vi "Untitled 4.vi"() -> ()   [LabVIEW 2016]
uses:
  <vilib>/addons/database/NI_Database_API.lvlib
  <vilib>/addons/database/Connection.llb/Conn Execute.vi
  <vilib>/addons/database/Recordset.llb/Rec Destroy - Connection.vi
panel:
  in  "POMPA":T1 {"DIAM mand [mm]" items=["--", "15", "20", "25", "27", "32", "40", "50", "65", "80", "100", "125", "150"]; "DIAM asp [mm]" items=["--", "15", "20", "25", "27", "32", "40", "50", "65", "80", "100", "125", "150"]; "MODELLO" items=["TECH 2", "TECH 3", "1", "2", "3", "4", "5", "1- FLOOR", "2- FLOOR", "2- VORTEX", "3- VORTEX", "2/20", "3/20", "4/40", "5/40", "TR 075", "30/50", "3SR2-15", "3SR2-22", "3SR2-30", "3SR2-43", "44/8", "4/9", "4/7", "4/14", "4/6 - 60Hz", "------", "12/6", "40/35", "55/35", "75/35", "40/65", "55/65", "75/65", "40/100", "50/100", "55/100", "15-50_st", "10-45", "15/50", "20/50", "30/50", "40/50", "50/50", "55/50", "TRm 1.1", "TRm 2.2", "18/18"]; "FAMIGLIA" items=["--", "TOP", "RX", "VX-71", "BC-71", "D", "VXC-71", "MC-71", "DC", "TRITUS", "VXC-80", "MC-80", "NK", "UP", "DAVIS", "4BLOCK", "4SR", "6SR", "TOP MULTI", "VXC4", "BC-100", "VX-100", "3SR", "4BLOCK", "MC4"]}
  in  "DATI GENERALI":T2 {"SCOPO" items=["--", "Audit", "Prototipo", "Campionatura", "Preserie", "Qualità", "Rientri", "Concorrenza"]; "NORMA DI RIFERIMENTO" items=["--", "0", "1", "2"]}
  in  "MOTORE":T3 {"GRADO IP" items=["--", "23", "44", "55", "68", "X4", "X5", "X8"]; "CLASSE ISOLAMENTO" items=["--", "B", "F", "H"]; "CONDENSATORE [uF,V]" items=["1", "2", "6.3", "8", "10", "12.5", "14", "16", "20", "25", "31.5", "35", "45", "------", "50"]; "Frequenza" items=["--", "50", "60", "Variabile"]; "FASI" items=["--", "Trifase", "Monofase"]; "MEC" items=["--", "56", "63", "71", "80", "90", "100", "112", "132", "160", "200", "250"]; "STATO" items=["--", "STD", "Prototipo", "Concorrenza"]}
  in  "CONDIZIONI DI PROVA":T4 {"COLLAUDATORE" items=["--", "CREMONESE G.PIETRO"]; "Fluido" items=["--", "Acqua"]}
  out "BOLLETTINO CARICATO":T5
  out "reversed":string
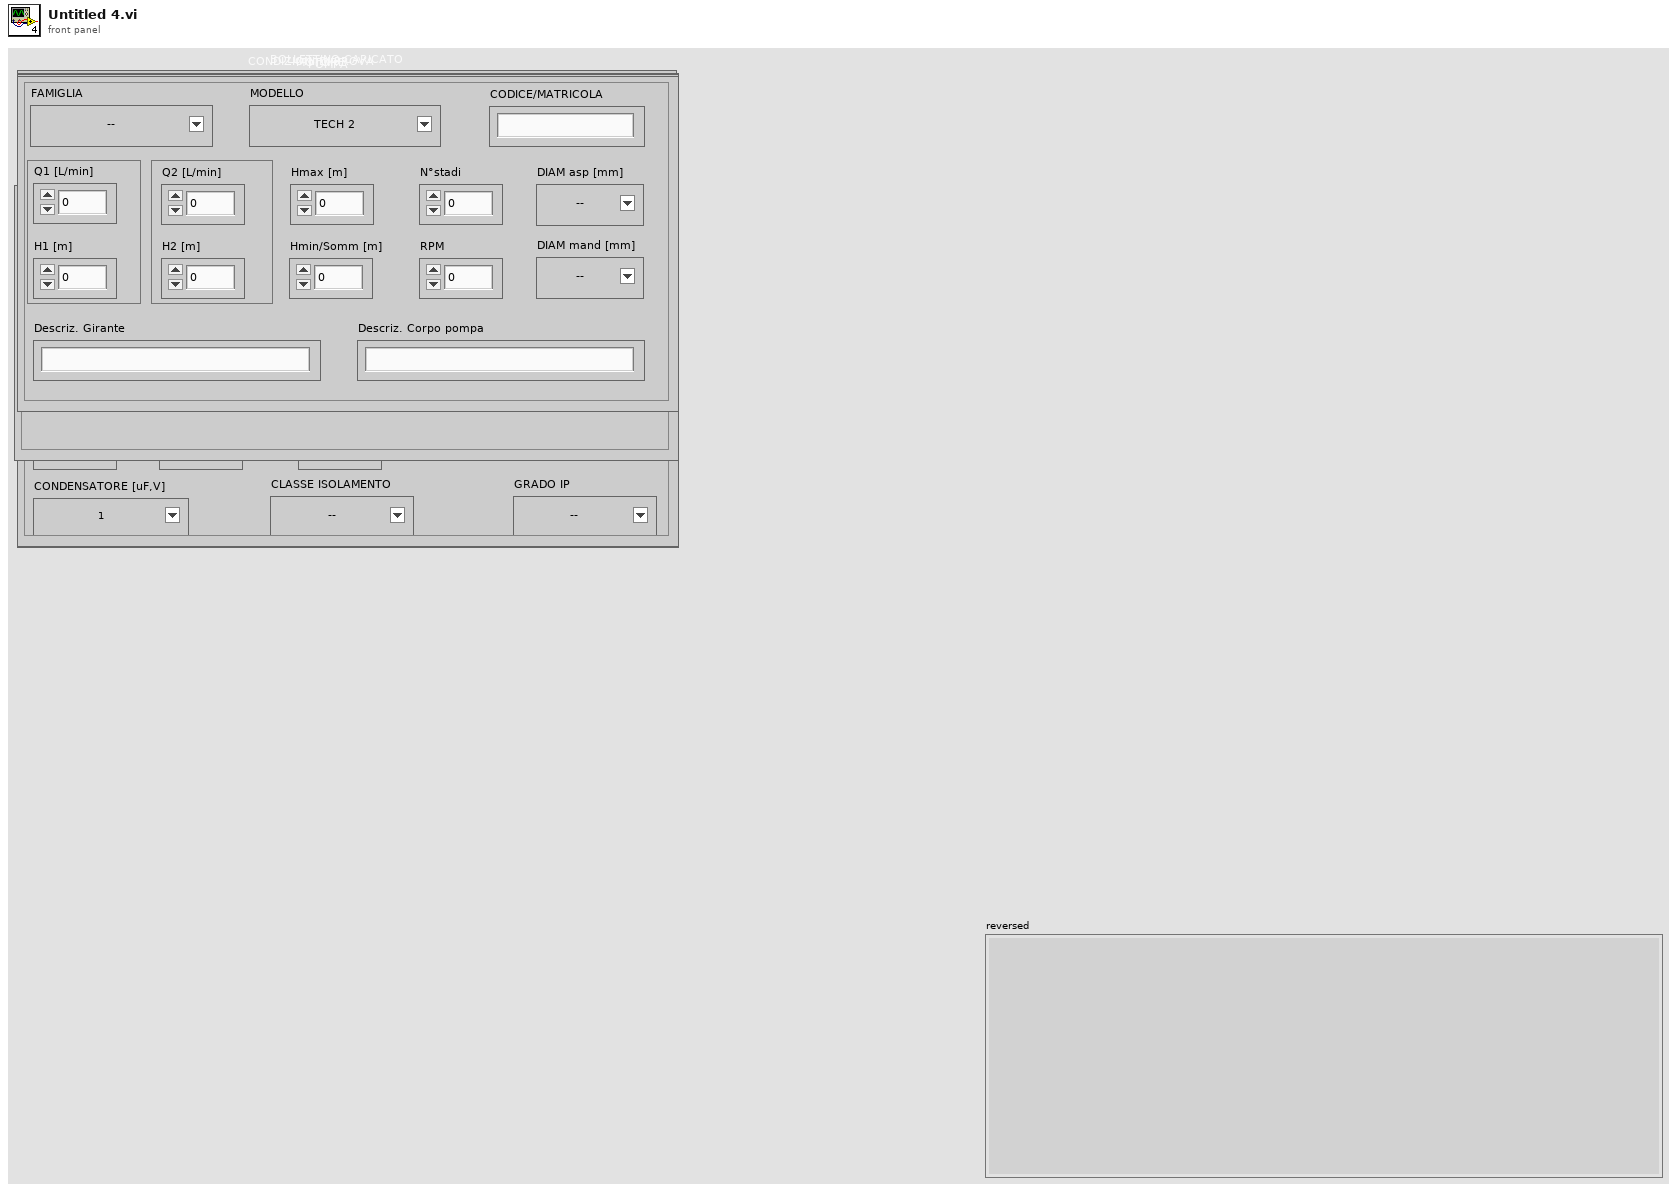
[diagram p1: front panel]
types:
  T1 = cluster{"FAMIGLIA":u16, "MODELLO":u16, "CODICE/MATRICOLA":string, "Q1 [L/min]":dbl, "Q2 [L/min] ":dbl, "H1 [m]":dbl, "H2 [m]":dbl, "Hmax [m]":dbl, "Hmin/Somm [m]":dbl, "RPM":dbl, "N°stadi":dbl, "DIAM asp [mm]":u16, "DIAM mand [mm]":u16, "Descriz. Girante":string, "Descriz. Corpo pompa":string}
  T2 = cluster{"NORMA DI RIFERIMENTO":u16, "SCOPO":u16, "ID PROGETTO":string, "N°ORDINE/PLP":string, "RIF/CLIENTE":string}
  T3 = cluster{"MODELLO E TIPO":string, "STATO":u16, "FILE TARATURA":string, "MEC":u16, "FASI":u16, "H pacco [mm]":dbl, "D est pacco[mm]":dbl, "D int pacco[mm]":dbl, "Tensione [V]":dbl, "Frequenza":u16, "N°poli":dbl, "RPM":dbl, "P2 nom [kW]":dbl, "P1 max [kW]":dbl, "I max [A]":dbl, "Rend max [%]":dbl, "CosFi":dbl, "CONDENSATORE [uF,V]":u16, "CLASSE ISOLAMENTO":u16, "GRADO IP":u16}
  T4 = cluster{"Trasd. P mandata":string, "Trasd. P aspirazione":string, "Dislivello trasd. P [m]":dbl, "Misuratore di Portata":string, "Rapporto TA":string, "Fluido":u16, "Temperatura fluido [°C]":string, "Massa volumica [kg/m3]":string, "Tensione vapore":string, "Tambiente [°C]":dbl, "Pbarometrica[Pa]":dbl, "Tensione di prova [V]":dbl, "Frequenza di prova [Hz]":dbl, "COLLAUDATORE":u16, "NOTE":string, "Set valvole tabella 1":string, "Set valvole tabella 2":string, "Set valvole tabella 3":string}
  T5 = cluster{"BANCO":string, "ANNO":string, "PROGRESSIVO":string, "TIPO PROVA":string, "PROVA SPECIALE ?":string, "DATA":string}
  T6 = cluster{"BOLLETTINO CARICATO":refnum<vi>, "DATI GENERALI":refnum<vi>, "POMPA":refnum<vi>, "MOTORE":refnum<vi>, "CONDIZIONI DI PROVA":refnum<vi>}
  T7 = typedef "NI_Database_API.lvlib/Conn ObjectReference.ctl" = refnum<k1>
  T8 = typedef "NI_Database_API.lvlib/Rec ObjectReference.ctl" = refnum<k1>
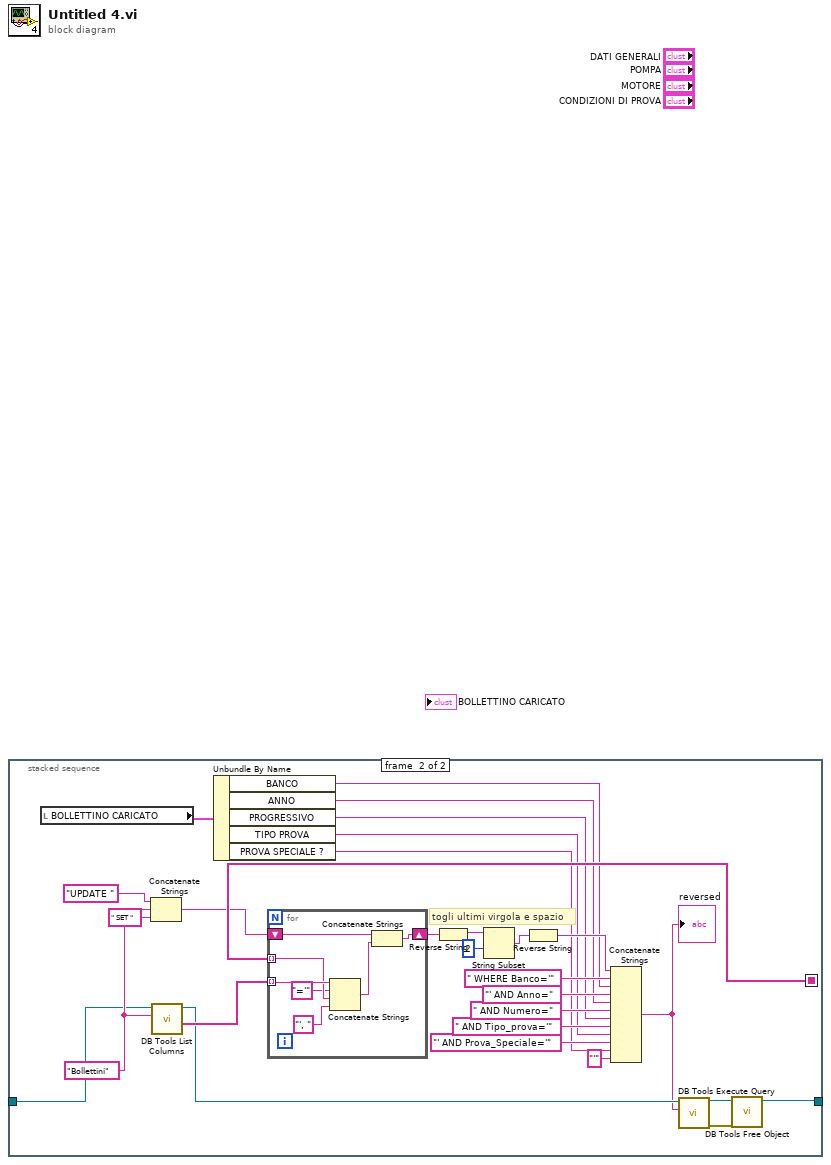
[diagram p0: block diagram]
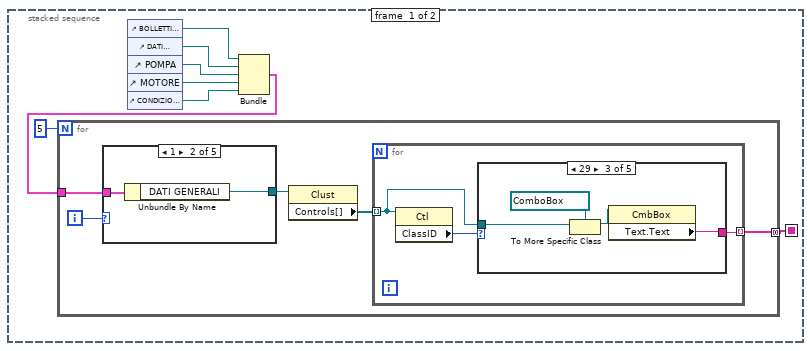
[diagram p2: hidden frame]
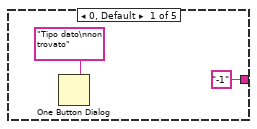
[diagram p3: hidden frame]
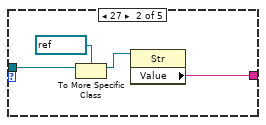
[diagram p4: hidden frame]
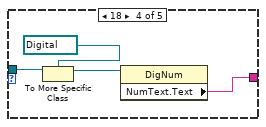
[diagram p5: hidden frame]
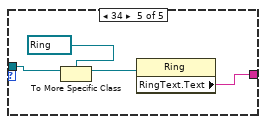
[diagram p6: hidden frame]
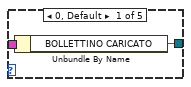
[diagram p7: hidden frame]
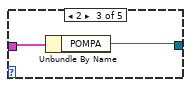
[diagram p8: hidden frame]
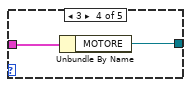
[diagram p9: hidden frame]
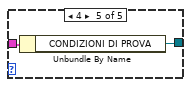
[diagram p10: hidden frame]
diagram:
  n1 = stacked-sequence {
    seq-local: [w1 _] -> [_ w70]
    tunnel: _ -> [_ w63]
    tunnel: [_ w48] -> _
    frame #0 {
      n2 = control-ref of="BOLLETTINO CARICATO"() -> (w3:refnum<vi>)
      n3 = control-ref of="DATI GENERALI"() -> (w4:refnum<vi>)
      n4 = control-ref of="POMPA"() -> (w5:refnum<vi>)
      n5 = control-ref of="MOTORE"() -> (w6:refnum<vi>)
      n6 = control-ref of="CONDIZIONI DI PROVA"() -> (w7:refnum<vi>)
      n7 = Bundle("BOLLETTINO CARICATO"=w3, "DATI GENERALI"=w4, "POMPA"=w5, "MOTORE"=w6, "CONDIZIONI DI PROVA"=w7) -> (w8:T6)  [unwired: 1 in]
      n8 = for {
        N: 5 -> [_]
        tunnel: w8 -> [w13]
        tunnel: [w9] -> w1 mode=concatenating
        i -> [w12]
        n9 = case shown="1" w12 {
          tunnel: w13 -> [w36 w38 w40 w42 w44]
          tunnel: [w35 w37 w39 w41 w43] -> w10
          frame 0, Default {
            n10 = Unbundle By Name(w36) -> ("BOLLETTINO CARICATO"=w35:refnum<vi>)
          }
          frame 1 {
            n11 = Unbundle By Name(w38) -> ("DATI GENERALI"=w37:refnum<vi>)
          }
          frame 2 {
            n12 = Unbundle By Name(w40) -> ("POMPA"=w39:refnum<vi>)
          }
          frame 3 {
            n13 = Unbundle By Name(w42) -> ("MOTORE"=w41:refnum<vi>)
          }
          frame 4 {
            n14 = Unbundle By Name(w44) -> ("CONDIZIONI DI PROVA"=w43:refnum<vi>)
          }
        }
        n15 = property class="Clust"(reference=w10) -> ("Controls[]"=w11:refnum<vi>[])  [unwired: 1 in, 2 out]
        n16 = for {
          tunnel: w11 -> [w15] mode=indexing
          tunnel: [w14] -> w9 mode=indexing
          n17 = property class="Ctl"(reference=w15) -> ("ClassID"=w16:u32)  [unwired: 1 in, 2 out]
          n18 = case shown="29" w16 {
            tunnel: w15 -> [_ w21 w24 w30 w33]
            tunnel: ["-1" ("RingText.Text") w19 w23 w27 w31] -> w14
            frame 0, Default {
              n19 = One Button Dialog(message="Tipo dato\nnon trovato") -> ()  [unwired: 1 in, 1 out]
            }
            frame 27 {
              n20 = To More Specific Class(target class=refnum<vi> refnum ("String"), reference=w21) -> (specific class reference=w20:refnum<vi>)  [unwired: 1 in, 1 out]
              n21 = property class="Str"(reference=w20) -> ("Value"=w19:string)  [unwired: 1 in, 2 out]
            }
            frame 29 {
              n22 = To More Specific Class(target class=refnum<vi> refnum ("String"), reference=w24) -> (specific class reference=w25:refnum<vi>)  [unwired: 1 in, 1 out]
              n23 = property class="CmbBox"(reference=w25) -> ("Text.Text"=w23:string)  [unwired: 1 in, 2 out]
            }
            frame 18 {
              n24 = To More Specific Class(target class=refnum<vi> refnum ("Numeric Control"), reference=w30) -> (specific class reference=w28:refnum<vi>)  [unwired: 1 in, 1 out]
              n25 = property class="DigNum"(reference=w28) -> ("NumText.Text"=w27:string)  [unwired: 1 in, 2 out]
            }
            frame 34 {
              n26 = To More Specific Class(target class=refnum<vi> refnum ("Menu Ring"), reference=w33) -> (specific class reference=w32:refnum<vi>)  [unwired: 1 in, 1 out]
              n27 = property class="Ring"(reference=w32) -> ("RingText.Text"=w31:string)  [unwired: 1 in, 2 out]
            }
          }
        }
      }
    }
    frame #1 {
      w72 = "Bollettini" ("table")
      # "togli ultimi virgola e spazio"
      n28 = local read "BOLLETTINO CARICATO"() -> (w60:T5)
      n29 = Concatenate Strings("UPDATE " ("table"), w72, " SET " ("string")) -> (w68:string)
      n30 = call <vilib>:"DB Tools List Columns.vi"("table"=w72, "connection reference"=w63) -> ("columns"=w71:string[], "connection reference out"=w50:T7)  [unwired: 2 in, 2 out]
      n31 = Unbundle By Name(w60) -> ("BANCO"=w59:string, "ANNO"=w57:string, "PROGRESSIVO"=w55:string, "TIPO PROVA"=w53:string, "PROVA SPECIALE ?"=w51:string)
      n32 = for {
        tunnel: w71 -> [w80] mode=indexing
        tunnel: w70 -> [w79] mode=indexing
        shift-right: [w75] -> w67
        shift-left: w68 -> [w77]
        n33 = Concatenate Strings(w80, "='" ("string"), w79, "', " ("string")) -> (w76:string)
        n34 = Concatenate Strings(w77, w76) -> (w75:string)
      }
      n35 = Reverse String(1:w67) -> (0:w66:string)
      n36 = String Subset(string=w66, offset (0)=2) -> (substring=w64:string)  [unwired: 1 in]
      n37 = Reverse String(1:w64) -> (0:w62:string)
      n38 = Concatenate Strings(w62, " WHERE Banco='" ("string"), w59, "' AND Anno=" ("string"), w57, " AND Numero=" ("string"), w55, " AND Tipo_prova='" ("string"), w53, "' AND Prova_Speciale='" ("string"), w51, "'" ("string")) -> (w47:string)
      "reversed" <- w47
      n39 = call-poly <vilib>:"DB Tools Execute Query.vi"("SQL query"=w47, "connection reference"=w50) -> ("error out"=w46:errorcluster, "recordset reference"=w49:T8)  [unwired: 6 in]
      n40 = call-poly <vilib>:"DB Tools Free Object.vi"("error in (no error)"=w46, "recordset reference"=w49) -> ("connection reference"=w48:T7)  [unwired: 8 in, 1 out]
    }
  }
